vi "project item dispatcher.vi"(4 "Export Diagram":bool, 6 "Create Captions":bool=TRUE, 8 "error in (no error)":errorcluster, 10 "String Files Root":path, 11 "ProjectItem in":refnum<vi>) -> (0 "error out":errorcluster)   [LabVIEW 2022 SP3]
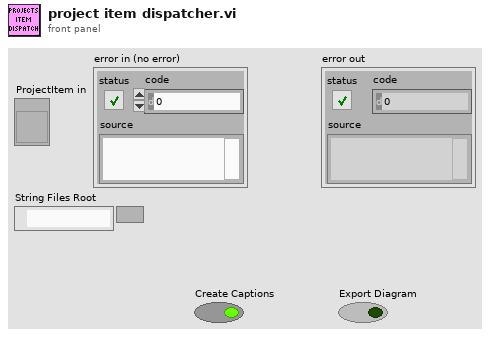
[diagram p1: front panel]
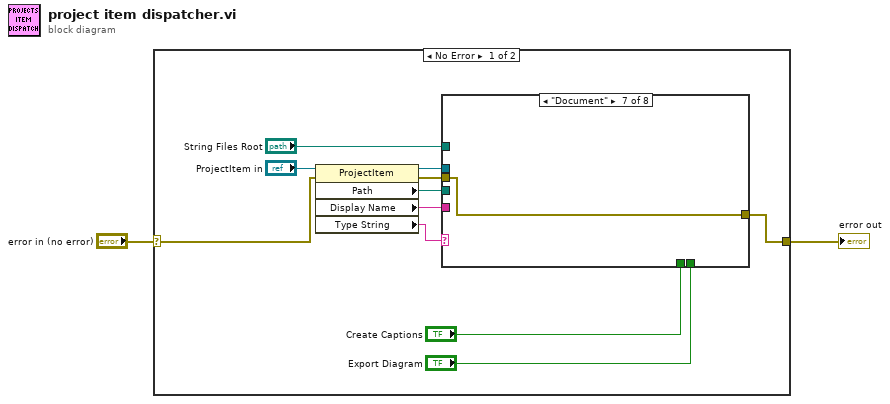
[diagram p0: block diagram]
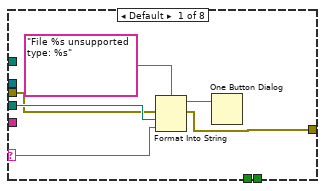
[diagram p2: hidden frame]
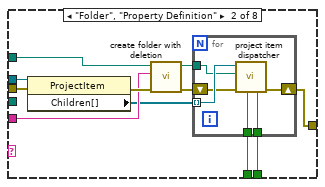
[diagram p3: hidden frame]
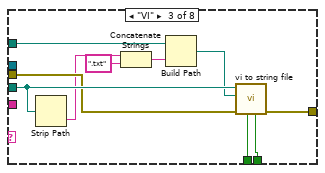
[diagram p4: hidden frame]
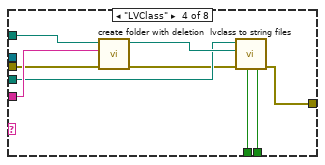
[diagram p5: hidden frame]
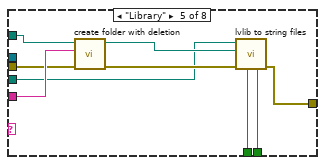
[diagram p6: hidden frame]
diagram:
  n1 = case shown="No Error" "error in (no error)" {
    selector: "error in (no error)" -> [w3 w68]
    tunnel: [w6 w68] -> w2
    frame No Error {
      n2 = property class="ProjectItem"(reference="ProjectItem in", error in=w3) -> (reference out=w4:refnum<vi>, error out=w7:errorcluster, "Path"=w12:path, "Display Name"=w5:string, "Type String"=w11:string)
      n3 = case shown="\"Document\"" w11 {
        selector: w11 -> [w16 _ _ _ _ _ _ _]
        tunnel: w12 -> [w17 _ w46 w52 w57 _ _ _]
        tunnel: "String Files Root" -> [_ w27 w45 w55 w64 _ _ _]
        tunnel: "Create Captions" -> [_ w22 w44 w49 w59 _ _ _]
        tunnel: "Export Diagram" -> [_ w21 w43 w48 w58 _ _ _]
        tunnel: w7 -> [w15 w29 w42 w47 w62 w65 w66 w67]
        tunnel: [w14 w20 w41 w50 w56 w65 w66 w67] -> w6
        tunnel: w5 -> [_ w26 _ w54 w63 _ _ _]
        tunnel: w4 -> [_ w30 _ _ _ _ _ _]
        frame Default {
          n4 = Format Into String(format string="File %s unsupported type: %s", error in=w15, w17, w16) -> (resulting string=w18:string, error out=w14:errorcluster)  [unwired: 1 in]
          n5 = One Button Dialog(message=w18) -> ()  [unwired: 1 in, 1 out]
        }
        frame "Folder", "Property Definition" {
          n6 = property class="ProjectItem"(reference=w30, error in=w29) -> (error out=w28:errorcluster, "Children[]"=w25:refnum<vi>[])  [unwired: 1 out]
          n7 = call "create folder with deletion.vi"("error in (no error)"=w28, "Folder Name"=w26, "Root path"=w27) -> ("error out"=w23:errorcluster, "created path"=w24:path)  [unwired: 7 in]
          n8 = for {
            tunnel: w25 -> [w36] mode=indexing
            tunnel: w24 -> [w35]
            shift-right: [w33] -> w20
            shift-left: w23 -> [w34]
            tunnel: w22 -> [w32]
            tunnel: w21 -> [w31]
            n9 = call "project item dispatcher.vi"("Export Diagram"=w31, "Create Captions"=w32, "error in (no error)"=w34, "String Files Root"=w35, "ProjectItem in"=w36) -> ("error out"=w33:errorcluster)  [unwired: 6 in]
          }
        }
        frame "VI" {
          n10 = Strip Path(path=w46) -> (name=w40:string)  [unwired: 1 out]
          n11 = Concatenate Strings(w40, ".txt" ("string")) -> (w39:string)
          n12 = Build Path(base path=w45, name or relative path=w39) -> (appended path=w37:path)
          n13 = call "vi to string file.vi"("Export Diagram"=w43, "Create Captions"=w44, "error in (no error)"=w42, "String File Path in"=w37, "VI Path in"=w46) -> ("error out"=w41:errorcluster)  [unwired: 4 in, 2 out]
        }
        frame "LVClass" {
          n14 = call "create folder with deletion.vi"("error in (no error)"=w47, "Folder Name"=w54, "Root path"=w55) -> ("error out"=w51:errorcluster, "created path"=w53:path)  [unwired: 7 in]
          n15 = call "lvclass to string files.vi"("Export Diagram"=w48, "Create Captions"=w49, "error in (no error)"=w51, "Class String Files Root"=w53, "lvclass Path"=w52) -> ("error out"=w50:errorcluster)  [unwired: 6 in]
        }
        frame "Library" {
          n16 = call "create folder with deletion.vi"("error in (no error)"=w62, "Folder Name"=w63, "Root path"=w64) -> ("error out"=w61:errorcluster, "created path"=w60:path)  [unwired: 7 in]
          n17 = call "lvlib to string files.vi"("Export Diagram"=w58, "Create Captions"=w59, "error in (no error)"=w61, "Library String Files Root"=w60, "lvlib Path"=w57) -> ("error out"=w56:errorcluster)  [unwired: 6 in]
        }
        frame "Dependencies" {
        }
        frame "Document" {
        }
        frame "Build" {
        }
      }
    }
    frame Error {
    }
  }
  "error out" <- w2
